vi "get corrected trace.vi"(8 "Trace 2D array":dbl[][](array[numeric]), 11 "Transducer 2D array":dbl[][](array[numeric])) -> (1 "yi":dbl[](array[numeric]) format="%_6g", 2 "xi used":dbl[](array[numeric]) format="%_6g", 3 "x+y":dbl[][](array[numeric]))   [LabVIEW 2016]
doc: "get corrected trace by interpolating Y value on top of transducer array,"
uses:
  <vilib>/gmath/NI_Gmath.lvlib
panel:
  out "Trace amplitude":dbl[](array[numeric])
  out "Trace Frequency":dbl[](array[numeric])
  out "XY Graph":cluster{"xi used":dbl[], dbl[]}(graph)
  out "Transducer factor":dbl[](array[numeric])
  out "Transducer Frequency":dbl[](array[numeric])
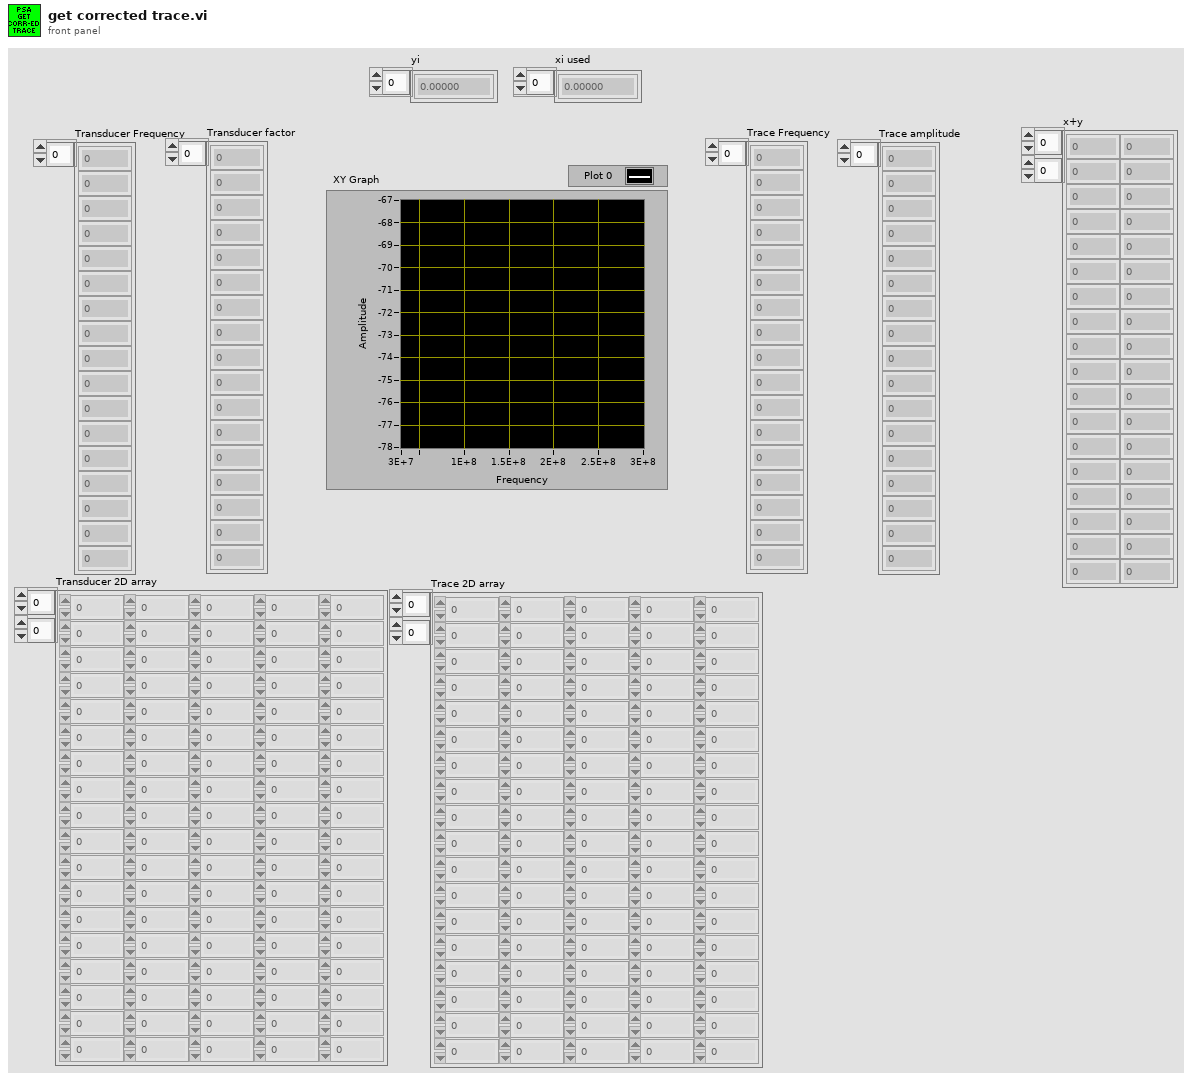
[diagram p1: front panel]
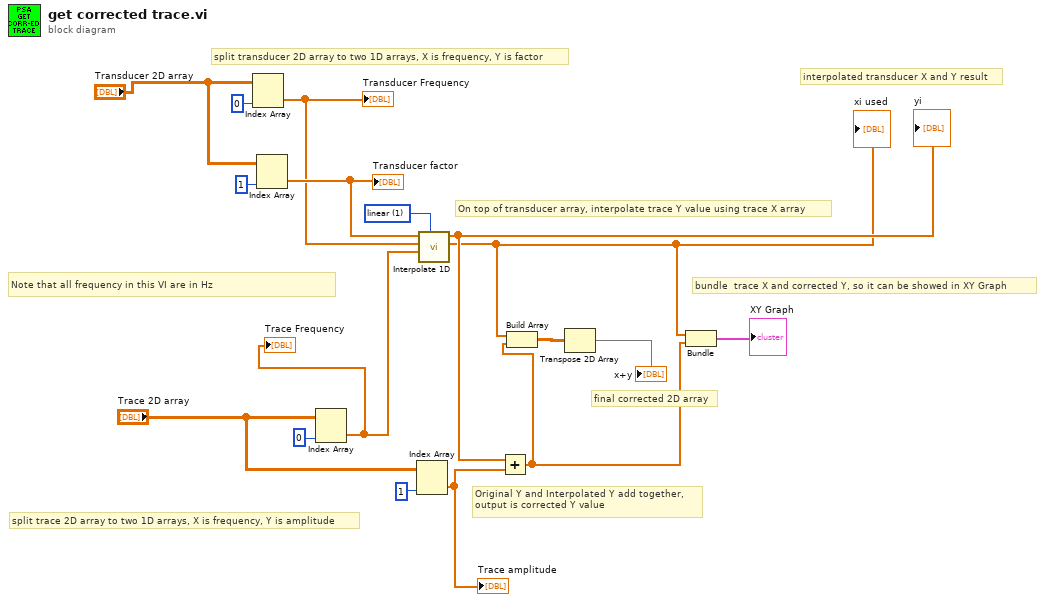
[diagram p0: block diagram]
diagram:
  w13 = 1 items=["nearest", "linear", "spline", "cubic Hermite", "Lagrange"] ("method")
  # "interpolated transducer X and Y result"
  # "Note that all frequency in this VI are in Hz"
  # "bundle  trace X and corrected Y, so it can be showed in XY Graph"
  # "final corrected 2D array"
  # "Original Y and Interpolated Y add together,\noutput is corrected Y value"
  # "On top of transducer array, interpolate trace Y value using trace X array"
  # "split trace 2D array to two 1D arrays, X is frequency, Y is amplitude"
  # "split transducer 2D array to two 1D arrays, X is frequency, Y is factor"
  n1 = Index Array(array="Transducer 2D array", index (col)=0 ("disabled index (col)")) -> (element=w14:dbl[])  [unwired: 1 in]
  "Transducer Frequency" <- w14
  n2 = Index Array(array="Transducer 2D array", index (col)=1 ("disabled index (col)")) -> (element=w15:dbl[])  [unwired: 1 in]
  "Transducer factor" <- w15
  n3 = Index Array(array="Trace 2D array", index (col)=0 ("disabled index (col)")) -> (element=w4:dbl[])  [unwired: 1 in]
  "Trace Frequency" <- w4
  n4 = Index Array(array="Trace 2D array", index (col)=1 ("disabled index (col)")) -> (element=w3:dbl[])  [unwired: 1 in]
  "Trace amplitude" <- w3
  n5 = call <vilib>:"Interpolate 1D.vi"("method"=w13, "xi"=w4, "X"=w14, "Y"=w15) -> ("xi used"=w7:dbl[], "yi"=w9:dbl[])  [unwired: 5 in, 1 out]
  "yi" <- w9
  "xi used" <- w7
  n6 = Add(x=w9, y=w3) -> (x+y=w5:dbl[])
  n7 = Build Array(w7, w5) -> (w12:dbl[][])
  n8 = Transpose 2D Array(2D array=w12) -> (transposed array=→"x+y":dbl[][])
  n9 = Bundle("xi used"=w7, w5) -> (→"XY Graph":cluster{"xi used":dbl[], dbl[]})  [unwired: 1 in]
